vi "SetPanelPosition__slk_mt.vi"(8 "error in (no error)":errorcluster, 11 "vi refnum in":refnum<vi>) -> (0 "error out":errorcluster)   [LabVIEW 2015, in "Lazyboots Menu Tool.lvlib"]
doc: "Sets VI panel to the right-bottom of primer monitor."
uses:
  <vilib>/SLK/Lazyboots Menu Tool/Library/Lazyboots Menu Tool.lvlib
panel:
  # "SetPanelPosition__slk_mt.vi\nSets VI panel to the right-bottom of primer monitor.\n\nNOTICE -- YOU MUST LEAVE THIS NOTICE IN PLACE.\n\nCopyright (c) 2011, LIANG LIU Shawn.Liu.cn@gmail.com\nAll rights reserved.\n\nRedistribution and use in source and binary forms, with or without modification, are permitted provided that the following conditions are met:\n-Redistributions of source code must retain the above copyright notice, this list of conditions and the following disclaimer.\n-Redistributions in binary form must reproduce the above copyright notice, this list of conditions and the following disclaimer in the documentation and/or other materials provided with the distribution.\n-Neither the name of the eLp nor the names of its contributors may be used to endorse or promote products derived from this software without specific prior written permission.\n\nTHIS SOFTWARE IS PROVIDED BY THE COPYRIGHT HOLDERS AND CONTRIBUTORS \"AS IS\" AND ANY EXPRESS OR IMPLIED WARRANTIES, INCLUDING, BUT NOT LIMITED TO, THE IMPLIED WARRANTIES OF MERCHANTABILITY AND FITNESS FOR A PARTICULAR PURPOSE ARE DISCLAIMED. IN NO EVENT SHALL THE COPYRIGHT HOLDER OR CONTRIBUTORS BE LIABLE FOR ANY DIRECT, INDIRECT, INCIDENTAL, SPECIAL, EXEMPLARY, OR CONSEQUENTIAL DAMAGES (INCLUDING, BUT NOT LIMITED TO, PROCUREMENT OF SUBSTITUTE GOODS OR SERVICES; LOSS OF USE, DATA, OR PROFITS; OR BUSINESS INTERRUPTION) HOWEVER CAUSED AND ON ANY THEORY OF LIABILITY, WHETHER IN CONTRACT, STRICT LIABILITY, OR TORT (INCLUDING NEGLIGENCE OR OTHERWISE) ARISING IN ANY WAY OUT OF THE USE OF THIS SOFTWARE, EVEN IF ADVISED OF THE POSSIBILITY OF SUCH DAMAGE."
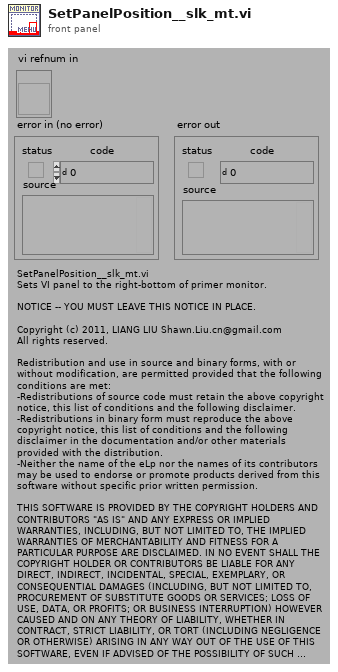
[diagram p1: front panel]
types:
  T1 = typedef "LVRectTypeDef.ctl" = cluster{"Left":i16, "Top":i16, "Right":i16, "Bottom":i16}
  T2 = cluster{"left":i16, "top":i16, "right":i16, "bottom":i16}
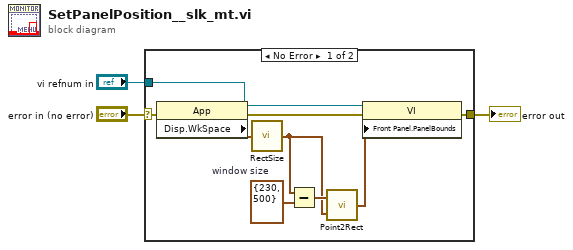
[diagram p0: block diagram]
diagram:
  n1 = case shown="No Error" "error in (no error)" {
    selector: "error in (no error)" -> [w5 w13]
    tunnel: "vi refnum in" -> [w8 _]
    tunnel: [w4 w13] -> w1
    frame No Error {
      w7 = cluster{"x":i16, "y":i16} {"x"=230, "y"=500}  # window size
      n2 = property class="App"(error in=w5) -> (error out=w6:errorcluster, "Disp.WkSpace"=w12:T1)  [unwired: 1 in, 1 out]
      n3 = call <vilib>:"RectSize.vi"("rect"=w12) -> ("point"=w9:cluster{"x":i16, "y":i16})
      n4 = Subtract(x=w9, y=w7) -> (x-y=w11:cluster{"x":i16, "y":i16})
      n5 = call <vilib>:"Point2Rect.vi"("point b"=w9, "point a"=w11) -> ("rect"=w10:T2)
      n6 = property class="VI"(reference=w8, error in=w6, "Front Panel.PanelBounds"=w10) -> (error out=w4:errorcluster)  [unwired: 1 out]
    }
    frame Error {
    }
  }
  "error out" <- w1
